vi "Init.vi"(3 "Container State":T6 caption="容器状态", 4 "Previous State":variant caption="前期状态", 5 "Previous Version":T5 caption="前期版本") -> (2 "Current State":T1={"method"=enum."None", "current color"=1, "available black position"=[], "available white position"=[], "Interactive Action"=refnum, "row"=0, "column"=0} caption="当前状态")   [LabVIEW 2011, in "Othello.xctl"]
uses:
  Othello.xctl
  State.ctl
  Control/Method Call.ctl
  Control/Pict Ring Chess.ctl
  Control/Interactive Action.ctl
  <vilib>/_xctls/Container State.ctl
  <vilib>/_xctls/Version.ctl
  <vilib>/_xctls/XControlSupport.lvlib
panel:
  in  "Default Indicator State":T1={"method"=enum."None", "current color"=1, "available black position"=[], "available white position"=[], "Interactive Action"=refnum, "row"=0, "column"=0} caption="默认显示控件状态"
  in  "Default Control State":T1={"method"=enum."None", "current color"=1, "available black position"=[], "available white position"=[], "Interactive Action"=refnum, "row"=0, "column"=0} caption="默认输入控件状态"
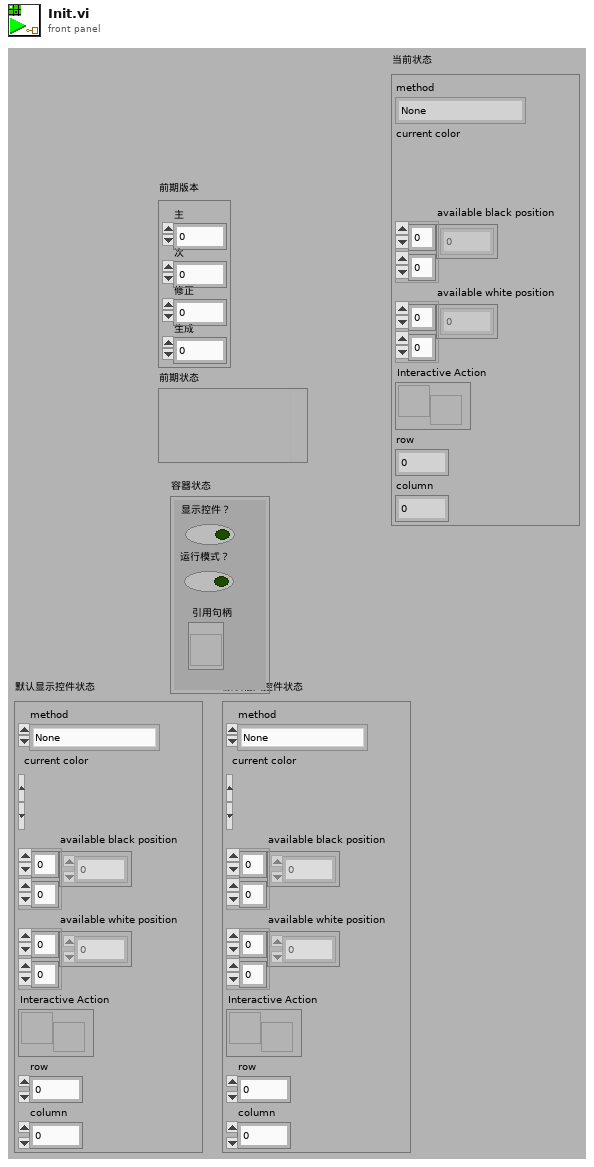
[diagram p1: front panel]
types:
  T1 = typedef "Othello.xctl/State.ctl" = cluster{"method":T2, "current color":T3, "available black position":i32[][], "available white position":i32[][], "Interactive Action":T4, "row":i32, "column":i32}
  T2 = typedef "Othello.xctl/Method Call.ctl" = enum16{"None", "New Game", "Play One"}
  T3 = typedef "Othello.xctl/Pict Ring Chess.ctl" = u16
  T4 = typedef "Othello.xctl/Interactive Action.ctl" = refnum<user-event>
  T5 = typedef "XControlSupport.lvlib/Version.ctl" = cluster{"Major":u16, "Minor":u16, "Fix":u16, "Build":u16}
  T6 = typedef "XControlSupport.lvlib/Container State.ctl" = cluster{"Indicator?":bool, "Run Mode?":bool, " Refnum":refnum<vi>}
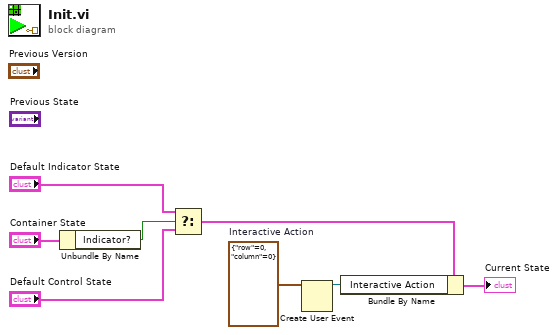
[diagram p0: block diagram]
diagram:
  w3 = cluster{"row":i32, "column":i32} {"row"=0, "column"=0}  # Interactive Action
  n1 = Unbundle By Name("Container State") -> ("Indicator?"=w5:bool)
  n2 = Select(t="Default Indicator State", s=w5, f="Default Control State") -> (s? t:f=w4:T1)
  n3 = Create User Event(user event datatype=w3) -> (user event=w2:refnum<user-event>)  [unwired: 1 in, 1 out]
  n4 = Bundle By Name(cluster=w4, "Interactive Action"=w2) -> (→"Current State":T1)
